vi "Check.vi"(8 "error in (no error)":errorcluster) -> (0 "error out":errorcluster, 3 "Pass? ( T)":bool=TRUE)   [LabVIEW 2020, in "WebServiceImporter.lvlib" / "Main Panel.lvlib" / "Input WSDL.lvlib"]
uses:
  <vilib>/Platform/WebService/Main Panel/Pages/Input WSDL/Input WSDL.lvlib
  <vilib>/Platform/WebService/Main Panel/Pages/Input WSDL/Events/Events.lvlib
  <vilib>/Platform/WebService/Main Panel/Events/Events.lvlib
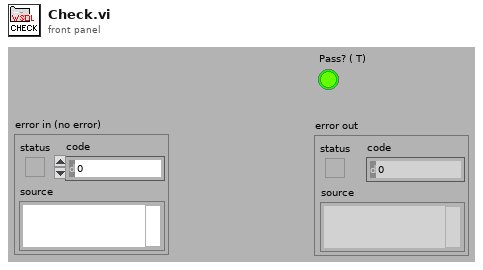
[diagram p1: front panel]
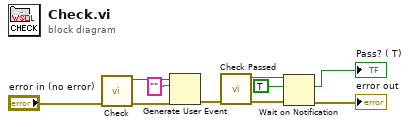
[diagram p0: block diagram]
diagram:
  n1 = call <vilib>:"Check.vi"("error in (no error)"="error in (no error)") -> ("error out"=w8:errorcluster, "user event (out)"=w9:refnum<user-event>)  [unwired: 9 in]
  n2 = Generate User Event(user event=w9, event data cluster="" ("event data"), error in=w8) -> (error out=w6:errorcluster)  [unwired: 1 in, 1 out]
  n3 = call <vilib>:"Check Passed.vi"("error in (no error)"=w6) -> ("error out"=w5:errorcluster, "notifier  (out)"=w4:refnum<notifier>)  [unwired: 9 in]
  n4 = Wait on Notification(notifier=w4, ignore previous (F)=TRUE, error in (no error)=w5) -> (notification=→"Pass? ( T)":bool, error out=→"error out":errorcluster)  [unwired: 1 in, 2 out]
